vi "SIM SourceType String to SrcType.vi"(1 "Source Type":string) -> (0 "Numeric":i32)   [LabVIEW 2017]
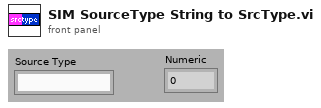
[diagram p1: front panel]
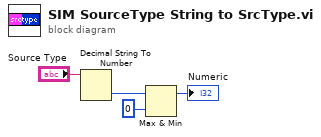
[diagram p0: block diagram]
diagram:
  n1 = Decimal String To Number(string="Source Type") -> (number=w1:i32)  [unwired: 3 out]
  n2 = Max & Min(x=w1, y=0) -> (max(x,y)=→"Numeric":i32)  [unwired: 1 out]
